vi "Sim Motors.vi"() -> ()   [LabVIEW 2012]
uses:
  <vilib>/Platform/TimedLoop/XDataNode/timing_clust.ctl
  <vilib>/Platform/TimedLoop/XDataNode/nitl_modes.ctl
  <vilib>/Platform/TimedLoop/XDataNode/wakeup.ctl
  <vilib>/robotics/Steering/Wheel/Wheel Parameters.ctl
  <vilib>/robotics/Steering/Wheel/Rotation Direction.ctl
  <vilib>/robotics/Simulator/Interface/Simulator References/Get Joint Reference (Hinge).vi
  <vilib>/robotics/Steering/Fixed Wheel/Create Fixed Wheel.vi
  <vilib>/robotics/Steering/Steering Frame/Create User Defined Steering Frame.vi
  <vilib>/robotics/Steering/Steering Frame/Apply Steering Frame Velocity to Motors.vi
  <vilib>/Platform/TimedLoop/XDataNode/XDataNode.xnode
  <vilib>/robotics/Steering/Create Steering Frame/NI_Robotics_Create Steering Frame.xnode
  <vilib>/robotics/Steering/Class Type Definitions/Steering Frame.ctl
  <vilib>/robotics/Steering/Steering Frame/NI_Robotics_Steering Frame.lvclass
  <vilib>/robotics/Steering/Class Type Definitions/NI_Robotics_Steering Class Types.lvlib
  <vilib>/Platform/TimedLoop/XDataNode/XDNodeRunTimeDep.lvlib
  <resource>/objmgr/LVODE.rc
  <vilib>/robotics/Simulator/NI_Robotics_Simulator.lvlib
  <vilib>/robotics/Steering/Fixed Wheel/NI_Robotics_Fixed Wheel.lvclass
  <vilib>/robotics/Steering/Wheel/NI_Robotics_Wheel.lvclass
panel:
  out "Telemetry":T1={"Voltage"={0.0, 0.0, 0.0}, "Encoder Speed"={0, 0}, "Temps"={"IC Temp (C)"=0, "Ch1 Temp (C)"=0, "Ch2 Temp (C)"=0}, "Current"={0.0, 0.0, 0.0, 4.6238981750249924e+36}} {"Current" scale=0.0..16.0; "Temps"."IC Temp (C)" scale=0.0..150.0; "Temps"."Ch1 Temp (C)" scale=0.0..150.0; "Temps"."Ch2 Temp (C)" scale=0.0..150.0; "Encoder Speed" scale=-100.0..100.0; "Voltage" scale=8.0..14.0}
  in  "error in":errorcluster
  out "error out":errorcluster
  in  "stop?":bool
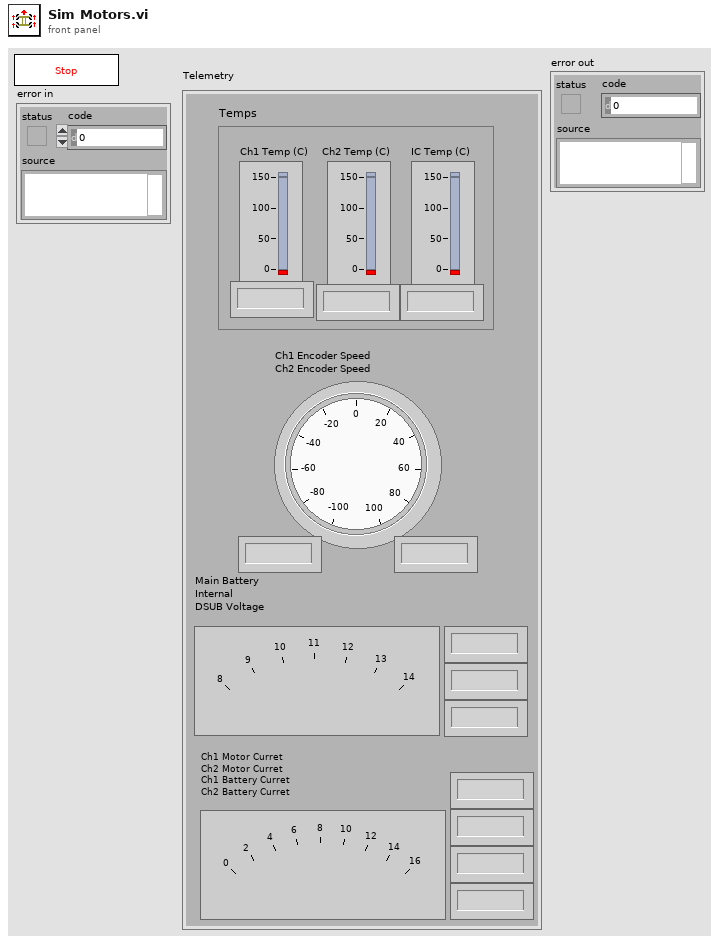
[diagram p1: front panel]
types:
  T1 = cluster{"Voltage":cluster{sgl, sgl, sgl}, "Encoder Speed":cluster{i32, i32}, "Temps":cluster{"IC Temp (C)":i32, "Ch1 Temp (C)":i32, "Ch2 Temp (C)":i32}, "Current":cluster{dbl, dbl, dbl, dbl}}
  T2 = cluster{"Robot":string, "Sensors":string[], "Joints":string[], "Actuators":string[], "Robot Components":string[]}[]
  T3 = cluster{"Robot":string, "Sensors":string[], "Joints":string[], "Actuators":string[], "Robot Components":string[]}
  T4 = typedef "NI_Robotics_Steering Class Types.lvlib/Steering Frame.ctl" = refnum<class "NI_Robotics_Steering Frame.lvclass">
  T5 = typedef "XDNodeRunTimeDep.lvlib/timing_clust.ctl" = cluster{"Expected End [f-1]":u64, "Actual End [f-1]":u64, "Finished Late? [f-1]":bool, "Expected End [i-1]":u64, "Actual End [i-1]":u64, "Finished Late? [i-1]":bool, "Expected Start [i]":u64, "Actual Start [i]":u64, "Expected Start [f]":u64, "Actual Start [f]":u64, "Source Name":string, "Structure Name":string, "Period":i64, "Deadline":i64, "Offset":i64, "Start":i64, "Priority":i32, "Timeout":i32, "Mode":T6, "Wakeup Reason":T7, "Error":errorcluster, "Source Type":string, "Secondary Source Type":string, "Global End Time":u64, "Global Start Time":u64, "Frame Duration":u64, "Iteration Duration":u64, "Assigned CPU":i32, "I/O Scan Engine Mode":u32}
  T6 = typedef "XDNodeRunTimeDep.lvlib/nitl_modes.ctl" = enum32{"No Change", "Process missed periods, maintain original phase", "Discard missed periods, maintain original phase", "Process missed periods, ignore original phase", "Discard missed periods, ignore original phase"}
  T7 = typedef "XDNodeRunTimeDep.lvlib/wakeup.ctl" = enum32{"Normal", "Aborted", "Asynchronous wakeup", "Timing source error", "Timed loop error", "Timeout"}
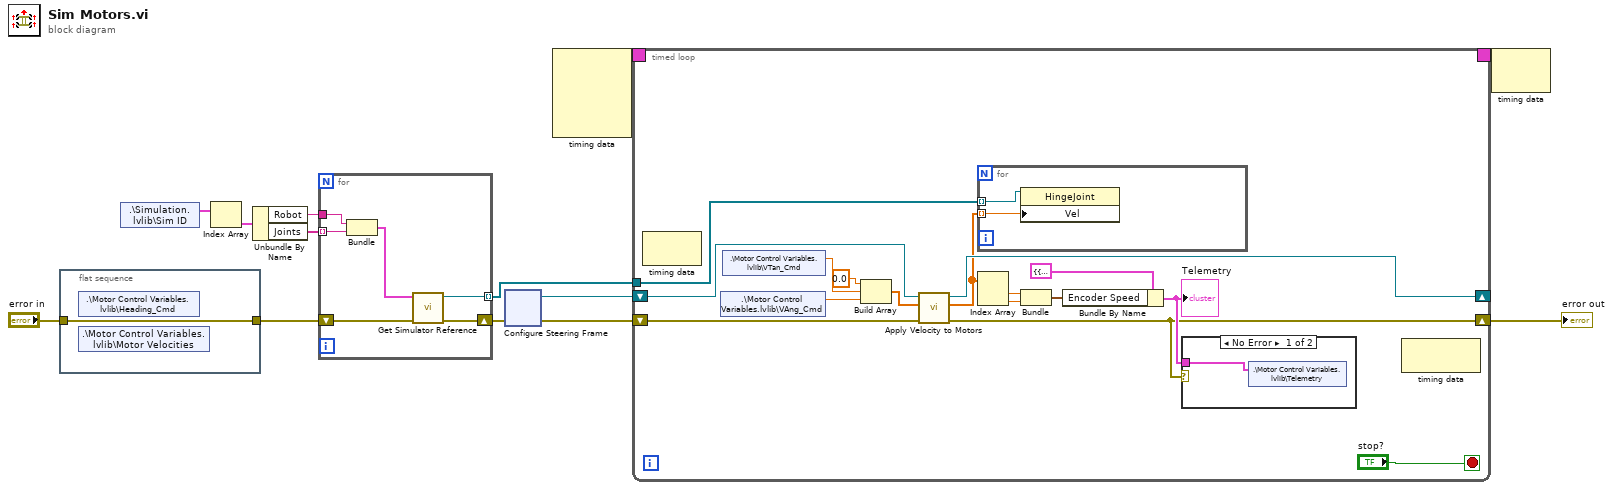
[diagram p0: block diagram]
diagram:
  n1 = flat-sequence {
    tunnel: [w14] -> w6
    tunnel: "error in" -> [w14]
    frame #0 {
      n2 = shared-variable ".\\Motor Control Variables.lvlib\\Heading_Cmd"() -> ()  [unwired: 1 in, 2 out]
      n3 = shared-variable ".\\Motor Control Variables.lvlib\\Motor Velocities"() -> ()  [unwired: 1 in, 2 out]
    }
  }
  n4 = shared-variable ".\\Simulation.lvlib\\Sim ID"() -> (w4:T2)  [unwired: 1 in, 1 out]
  n5 = Index Array(array=w4) -> (element=w3:T3)  [unwired: 1 in]
  n6 = Unbundle By Name(w3) -> ("Robot"=w2:string, "Joints"=w1:string[])
  n7 = for {
    tunnel: [w19] -> w7 mode=indexing
    shift-right: [w18] -> w5
    shift-left: w6 -> [w17]
    tunnel: w1 -> [w16] mode=indexing
    tunnel: w2 -> [w15]
    n8 = Bundle("Robot"=w15, w16) -> (w20:cluster{"Robot":string, string})  [unwired: 1 in]
    n9 = call-poly <vilib>:"Get Simulator Reference.vi"("error in (no error)"=w17, "robot joint ID"=w20) -> ("error out"=w18:errorcluster, "hinge joint ref"=w19:refnum<k20>)  [unwired: 8 in]
  }
  n10 = xnode ("Configure Steering Frame")("error in (no error)"=w5) -> ("steering frame out"=w10:T4, "error out"=w9:errorcluster)
  n11 = node-c288() -> (w13:T5)  [unwired: 4 in]
  n12 = timed-loop {
    timing: w13 -> [_]
    timing-out: [_] -> w12
    shift-right: [w34] -> _
    shift-left: w10 -> [w33]
    shift-right: [w23] -> w11
    shift-left: w9 -> [w32]
    tunnel: w7 -> [w22]
    stop <- "stop?" stop-if-true
    n13 = node-c288() -> ()  [unwired: 1 in, 1 out]
    n14 = shared-variable ".\\Motor Control Variables.lvlib\\VAng_Cmd"() -> (w29:dbl)  [unwired: 1 in, 1 out]
    n15 = shared-variable ".\\Motor Control Variables.lvlib\\VTan_Cmd"() -> (w30:dbl)  [unwired: 1 in, 1 out]
    n16 = Build Array(0.0 ("element"), w30, w29) -> (w36:dbl[])
    n17 = call-poly <vilib>:"Apply Velocity to Motors.vi"("error in (no error)"=w32, "steering frame velocity"=w36, "steering frame in"=w33) -> ("error out"=w23:errorcluster, "ccw motor velocity setpoints"=w21:dbl[], "steering frame out"=w34:T4)  [unwired: 4 in, 2 out]
    n18 = for {
      tunnel: w22 -> [w38] mode=indexing
      tunnel: w21 -> [w37] mode=indexing
      n19 = property on="Property Node 3" class="HingeJoint"(reference=w38, "Vel"=w37) -> ()  [unwired: 1 in, 2 out]
    }
    n20 = Index Array(array=w21) -> (element #1=w26:dbl, element #2=w25:dbl)  [unwired: 2 in]
    n21 = Bundle("Numeric"=w26, "Numeric"=w25) -> (w24:cluster{"Numeric":dbl, "Numeric":dbl})  [unwired: 1 in]
    n22 = Bundle By Name(cluster=T1 {"Voltage"={0.0, 0.0, 0.0}, "Encoder Speed"={0, 0}, "Temps"={"IC Temp (C)"=0, "Ch1 Temp (C)"=0, "Ch2 Temp (C)"=0}, "Current"={0.0, 0.0, 0.0, 0.0}} ("Telemetry"), "Encoder Speed"=w24) -> (w27:T1)
    "Telemetry" <- w27
    n23 = case shown="No Error" w23 {
      tunnel: w27 -> [w39 _]
      frame No Error {
        n24 = shared-variable ".\\Motor Control Variables.lvlib\\Telemetry"(w39) -> ()  [unwired: 1 in, 1 out]
      }
      frame Error {
      }
    }
    n25 = node-c288() -> ()  [unwired: 1 in, 1 out]
  }
  "error out" <- w11
  n26 = node-c288(w12) -> ()  [unwired: 1 out]
